vi "Variable Tree Update .vi"(8 "error in (no error)":errorcluster, 10 "Variable Tree":refnum<vi>, 11 "Project in":refnum<class "Project.lvclass">) -> (0 "error out":errorcluster, 3 "Project out":refnum<class "Project.lvclass">)   [LabVIEW 2015, in "Project.lvclass"]
uses:
  Project.lvclass
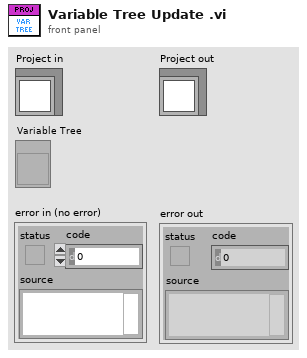
[diagram p1: front panel]
types:
  T1 = typedef "imagedata.ctl" = cluster{"image type":i32, "image depth":i32, "image":u8[], "mask":u8[], "colors":u32[], "Rectangle":cluster{"left":i16, "top":i16, "right":i16, "bottom":i16}}
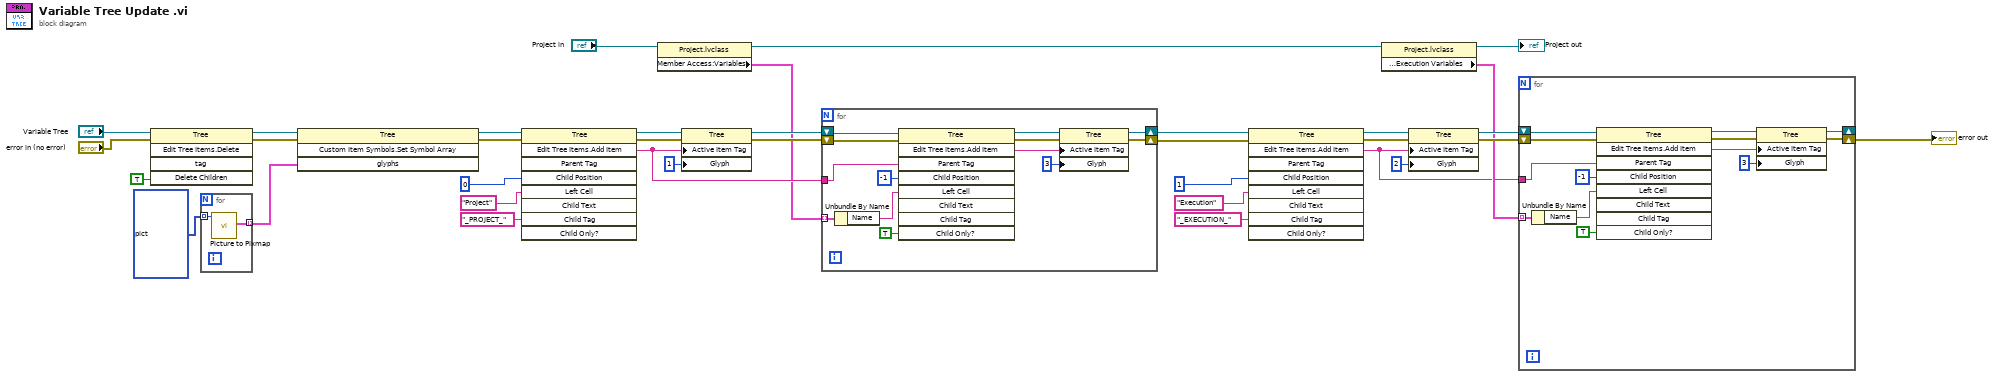
[diagram p0: block diagram]
diagram:
  n1 = invoke class="Tree" method="Edit Tree Items.Delete"(reference="Variable Tree", error in="error in (no error)", "Delete Children"=TRUE ("Delete Children?")) -> (reference out=w32:refnum<vi>, error out=w31:errorcluster)  [unwired: 2 in, 3 out]
  n2 = for {
    tunnel: picture[] [bytes[0], bytes[830], bytes[830], bytes[562]] -> [w37] mode=indexing
    tunnel: [w36] -> w29 mode=indexing
    n3 = call <vilib>:"Picture to Pixmap.vi"("picture"=w37) -> ("image data"=w36:T1)  [unwired: 9 in, 1 out]
  }
  n4 = invoke class="Tree" method="Custom Item Symbols.Set Symbol Array"(reference=w32, error in=w31, "glyphs"=w29) -> (reference out=w28:refnum<vi>, error out=w27:errorcluster)  [unwired: 1 in, 2 out]
  n5 = invoke class="Tree" method="Edit Tree Items.Add Item"(reference=w28, error in=w27, "Child Position"=0, "Left Cell"="Project", "Child Tag"="_PROJECT_") -> (reference out=w24:refnum<vi>, error out=w23:errorcluster, "Edit Tree Items:Add Item"=w11:string)  [unwired: 4 in, 6 out]
  n6 = property class="Project.lvclass"(reference="Project in") -> (reference out=w5:refnum<class "Project.lvclass">, "Member Access:Variables"=w10:cluster{"Name":string, "Value":variant}[])  [unwired: 1 in, 1 out]
  n7 = property class="Tree"(reference=w24, error in=w23, "Active Item Tag"=w11, "Glyph"=1) -> (reference out=w13:refnum<vi>, error out=w12:errorcluster)
  n8 = for {
    tunnel: w11 -> [w44]
    tunnel: w10 -> [w42] mode=indexing
    shift-right: [w39] -> w9
    shift-left: w13 -> [w46]
    shift-right: [w38] -> w8
    shift-left: w12 -> [w45]
    n9 = Unbundle By Name(w42) -> ("Name"=w41:string)
    n10 = invoke class="Tree" method="Edit Tree Items.Add Item"(reference=w46, error in=w45, "Parent Tag"=w44, "Child Position"=-1, "Left Cell"=w41, "Child Only?"=TRUE) -> (reference out=w47:refnum<vi>, error out=w48:errorcluster, "Edit Tree Items:Add Item"=w49:string)  [unwired: 3 in, 6 out]
    n11 = property class="Tree"(reference=w47, error in=w48, "Active Item Tag"=w49, "Glyph"=3) -> (reference out=w39:refnum<vi>, error out=w38:errorcluster)
  }
  n12 = invoke class="Tree" method="Edit Tree Items.Add Item"(reference=w9, error in=w8, "Child Position"=1, "Left Cell"="Execution", "Child Tag"="_EXECUTION_") -> (reference out=w19:refnum<vi>, error out=w20:errorcluster, "Edit Tree Items:Add Item"=w3:string)  [unwired: 4 in, 6 out]
  n13 = property class="Project.lvclass"(reference=w5) -> (reference out=→"Project out":refnum<class "Project.lvclass">, "Member Access:Execution Variables"=w4:cluster{"Name":string, "Value":variant}[])  [unwired: 1 in, 1 out]
  n14 = property class="Tree"(reference=w19, error in=w20, "Active Item Tag"=w3, "Glyph"=2) -> (reference out=w7:refnum<vi>, error out=w6:errorcluster)
  n15 = for {
    tunnel: w3 -> [w57]
    tunnel: w4 -> [w55] mode=indexing
    shift-right: [w52] -> _
    shift-left: w7 -> [w59]
    shift-right: [w51] -> w2
    shift-left: w6 -> [w58]
    n16 = Unbundle By Name(w55) -> ("Name"=w54:string)
    n17 = invoke class="Tree" method="Edit Tree Items.Add Item"(reference=w59, error in=w58, "Parent Tag"=w57, "Child Position"=-1, "Left Cell"=w54, "Child Only?"=TRUE) -> (reference out=w60:refnum<vi>, error out=w61:errorcluster, "Edit Tree Items:Add Item"=w62:string)  [unwired: 3 in, 6 out]
    n18 = property class="Tree"(reference=w60, error in=w61, "Active Item Tag"=w62, "Glyph"=3) -> (reference out=w52:refnum<vi>, error out=w51:errorcluster)
  }
  "error out" <- w2
